vi "getMethod.vi"(8 "error in (no error)":errorcluster, 11 "GraphSearch in":refnum<class "GraphSearch.lvclass">) -> (0 "error out":errorcluster, 2 "method":T1, 3 "GraphSearch out":refnum<class "GraphSearch.lvclass">)   [LabVIEW 2009, in "GraphSearch.lvclass"]
uses:
  GraphSearch.lvclass
  method.ctl
  GraphSearch.lvclass/GraphSearch.ctl
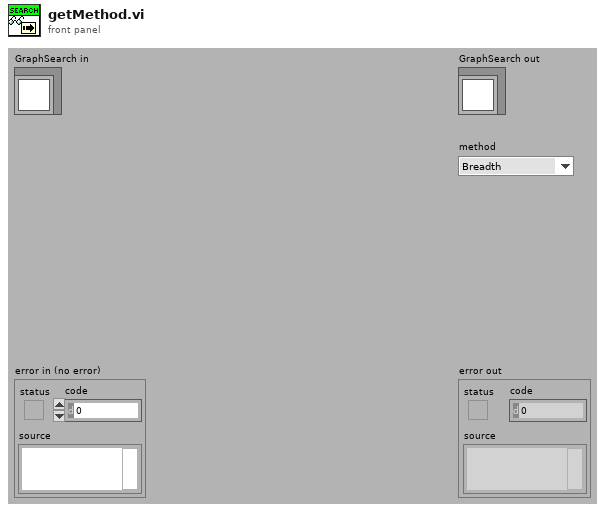
[diagram p1: front panel]
types:
  T1 = typedef "GraphSearch.lvclass/method.ctl" = enum16{"Breadth", "Heuristic", "Depth"}
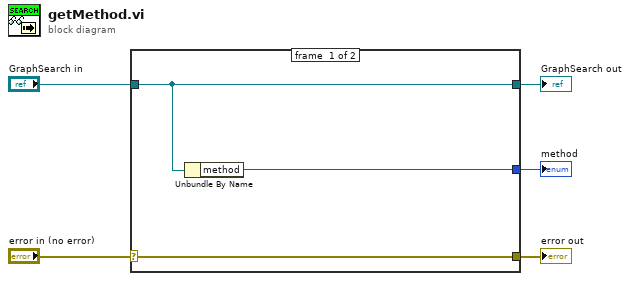
[diagram p0: block diagram]
diagram:
  n1 = case shown="No Error" "error in (no error)" {
    selector: "error in (no error)" -> [w8 w9]
    tunnel: [w8 w9] -> w4
    tunnel: [w7 w10] -> w2
    tunnel: "GraphSearch in" -> [w7 w10]
    tunnel: [w6 _] -> w1
    frame #0 {
      n2 = Unbundle By Name(w7) -> ("method"=w6:T1)
    }
    frame #1 {
    }
  }
  "error out" <- w4
  "GraphSearch out" <- w2
  "method" <- w1
